vi "RemoveDtProperty.vi"(11 "props in":T1[](array[typedef])) -> (3 "props out":T1[](array[typedef]))   [LabVIEW 2017, in "McsaDataEventCreator.lvlib"]
uses:
  <vilib>/addons/InsightCM/Devices/Shared/Mcsa/McsaDataEventCreator/McsaDataEventCreator.lvlib
  <vilib>/addons/InsightCM/MessageBus/Base/controls/KeyValuePair.ctl
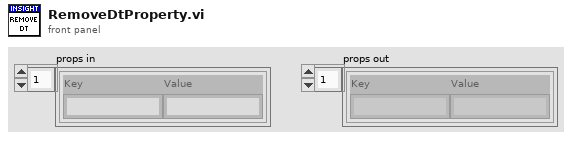
[diagram p1: front panel]
types:
  T1 = typedef "KeyValuePair.ctl" = cluster{"Key":string, "Value":string}
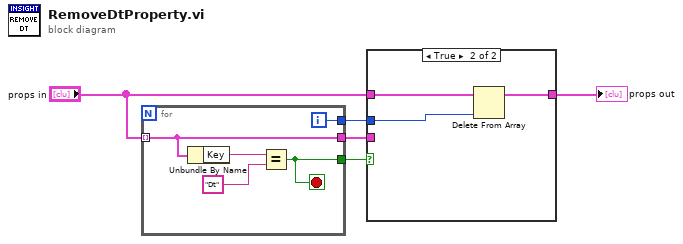
[diagram p0: block diagram]
diagram:
  n1 = for {
    tunnel: "props in" -> [w8] mode=indexing
    tunnel: [w9] -> w3
    tunnel: [w8] -> w4
    tunnel: [w7] -> w5
    i -> [w7]
    stop <- w9 stop-if-true
    n2 = Unbundle By Name(w8) -> ("Key"=w10:string)
    n3 = Equal?(x=w10, y="Dt" ("key")) -> (x = y?=w9:bool)
  }
  n4 = case shown="True" w3 {
    tunnel: w4 -> [_ _]
    tunnel: w5 -> [_ w13]
    tunnel: "props in" -> [w11 w14]
    tunnel: [w11 w12] -> w1
    frame False {
    }
    frame True {
      n5 = Delete From Array(array=w14, index=w13) -> (array with subset deleted=w12:T1[])  [unwired: 1 in, 1 out]
    }
  }
  "props out" <- w1
